vi "Set Digital Pin Mode.vi"(8 "Error In":errorcluster, 10 "Digtal Pin Modes":T1[](array[typedef]), 11 "LINX Device Config":T3) -> (0 "Error Out":errorcluster, 3 "LINX Device Config":T3)   [LabVIEW 2020, in "Device.lvlib"]
doc: "Configure digital I/O pins as inputs or outputs."
uses:
  Device.lvlib
  Type Defs/Error Type.ctl
  LMH-LINX.lvlib
  Type Defs/Interface.ctl
  Type Defs/Peripherals/Digital/Digital Pin Mode.ctl
  Type Defs/Peripherals/Digital/Digital Pin Configuration.ctl
  Type Defs/Channels.ctl
  Type Defs/TCP Config.ctl
  Type Defs/LINX Device Config.ctl
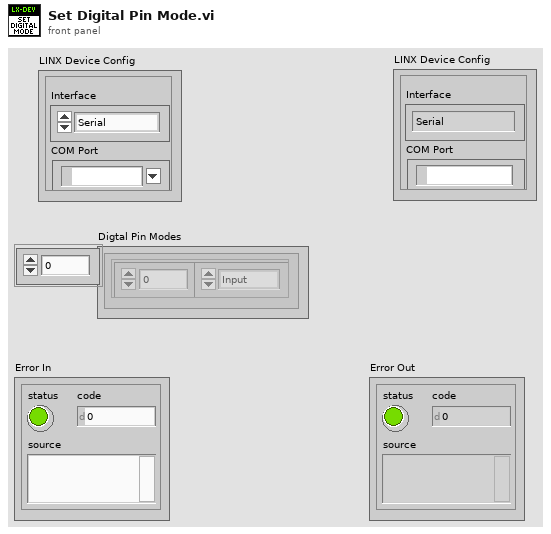
[diagram p1: front panel]
types:
  T1 = typedef "LMH-LINX.lvlib/Digital Pin Configuration.ctl" = cluster{"Pin Number":u8, "Digital Pin Mode":T2}
  T2 = typedef "LMH-LINX.lvlib/Digital Pin Mode.ctl" = enum8{"Input", "Output"}
  T3 = typedef "Device.lvlib/LINX Device Config.ctl" = cluster{"Interface":T4, "COM Port":refnum<visa-resource-name>, "TCP Configuration":T5, "Device Family":u8, "Device ID":u8, "Device Name":string, "TCP Ref":refnum<k5>, "Channels":T6}
  T4 = typedef "LMH-LINX.lvlib/Interface.ctl" = enum16{"Serial", "TCP"}
  T5 = typedef "Device.lvlib/TCP Config.ctl" = cluster{"IP Address":string, "Port":u16}
  T6 = typedef "LMH-LINX.lvlib/Channels.ctl" = cluster{"DI":u8[], "DO":u8[], "AI":u8[], "AO":u8[], "PWM":u8[], "QE":u8[], "UART":u8[], "I2C 2":u8[], "SPI":u8[], "CAN":u8[], "Servo":u8[], "AI Ref (V)":dbl, "AI Resolution (Bits)":u8, "AO Ref (V)":dbl, "AO Resolution (Bits)":u8}
  T7 = typedef "LMH-LINX.lvlib/Error Type.ctl" = enum16{"Unknown", "Timeout", "Corrupt Return Packet", "Unable To Connect", "Command Not Supported", "Channel DNE", "Invalid COM Config", "Firmware Version Mismatch", "myRIO Support", "CMD Specific Error", "Local IO Not Supported"}
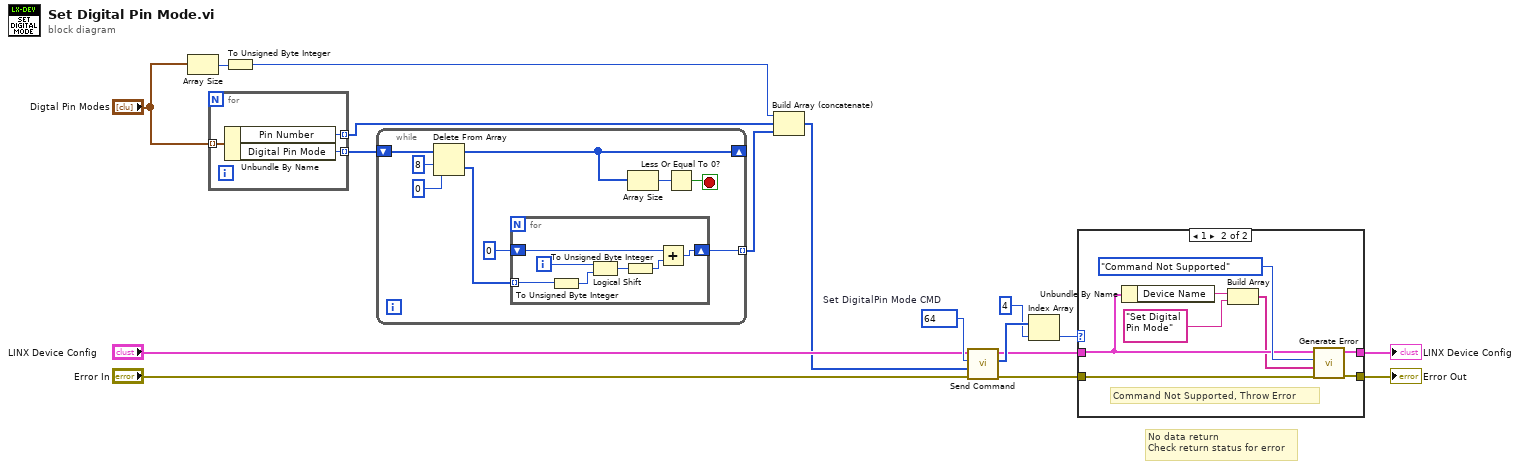
[diagram p0: block diagram]
diagram:
  w16 = u16 64  # Set DigitalPin Mode CMD
  # "No data return\nCheck return status for error"
  n1 = Array Size(array="Digtal Pin Modes") -> (size(s)=w12:i32)
  n2 = for {
    tunnel: "Digtal Pin Modes" -> [w20] mode=indexing
    tunnel: [w19] -> w13 mode=indexing
    tunnel: [w18] -> w14 mode=indexing
    n3 = Unbundle By Name(w20) -> ("Pin Number"=w19:u8, "Digital Pin Mode"=w18:T2)
  }
  n4 = To Unsigned Byte Integer(number=w12) -> (unsigned 8bit integer=w11:u8)
  n5 = while {
    shift-right: [w26] -> _
    shift-left: w14 -> [w29]
    tunnel: [w21] -> w1 mode=indexing
    stop <- w24 stop-if-true
    n6 = Delete From Array(array=w29, length=8 ("index"), index=0 ("length")) -> (deleted portion=w22:T2[], array with subset deleted=w26:T2[])
    n7 = for {
      shift-right: [w35] -> w21
      shift-left: u8 0 ("y") -> [w36]
      tunnel: w22 -> [w32] mode=indexing
      i -> [w30]
      n8 = To Unsigned Byte Integer(number=w32) -> (unsigned 8bit integer=w31:u8)
      n9 = Logical Shift(y=w30, x=w31) -> (x << y=w34:u8)
      n10 = To Unsigned Byte Integer(number=w34) -> (unsigned 8bit integer=w33:u8)
      n11 = Add(x=w36, y=w33) -> (x+y=w35:u8)
    }
    n12 = Array Size(array=w26) -> (size(s)=w25:i32)
    n13 = Less Or Equal To 0?(x=w25) -> (x <= 0?=w24:bool)
  }
  n14 = Build Array (concatenate)(w11, w13, w1) -> (w10:u8[])
  n15 = call "Send Command.vi"("Error In"="Error In", "ARGS"=w10, "CMD"=w16, "LINX Device Config"="LINX Device Config") -> ("Error Out"=w3:errorcluster, "Response"=w9:u8[], "LINX Device Config"=w5:T3)  [unwired: 4 in, 1 out]
  n16 = Index Array(array=w9, index=4) -> (element=w7:u8)
  n17 = case shown="1" w7 {
    tunnel: [w38 w44] -> w6
    tunnel: w5 -> [w38 w40]
    tunnel: [w37 w45] -> w4
    tunnel: w3 -> [w37 w46]
    frame 0, Default {
      # "Status OK"
    }
    frame 1 {
      # "Command Not Supported, Throw Error"
      n18 = Unbundle By Name(w40) -> ("Device Name"=w42:string)
      n19 = Build Array(w42, "Set Digital Pin Mode") -> (w39:string[])
      n20 = call "Generate Error.vi"("Error In"=w46, "Arguments"=w39, "Error Type"=Error_Type."Command Not Supported", "LINX Device Config"=w40) -> ("Error Out"=w45:errorcluster, "Dup LINX Device Config"=w44:T3)  [unwired: 6 in]
    }
  }
  "Error Out" <- w4
  "LINX Device Config" <- w6
